vi "GPX_speed_test.vi"() -> ()   [LabVIEW 2017]
uses:
  <vilib>/Analysis/NI_AALPro.lvlib
panel:
  in  "GPX File Path":path
  out "acceleration graph":cluster{timestamp[], dbl[]}[](graph)
  out "acc Integral speed":dbl[](array[numeric])
  out "gps mean speed":dbl format="%0.2f"
  out "distance [m]":dbl
  in  "elotlás [s]":dbl
  in  "Eltol":bool
  out "delta t [s]":dbl
  in  "stop":bool
  in  "reset":bool
  in  "binary path (use dialog)":path
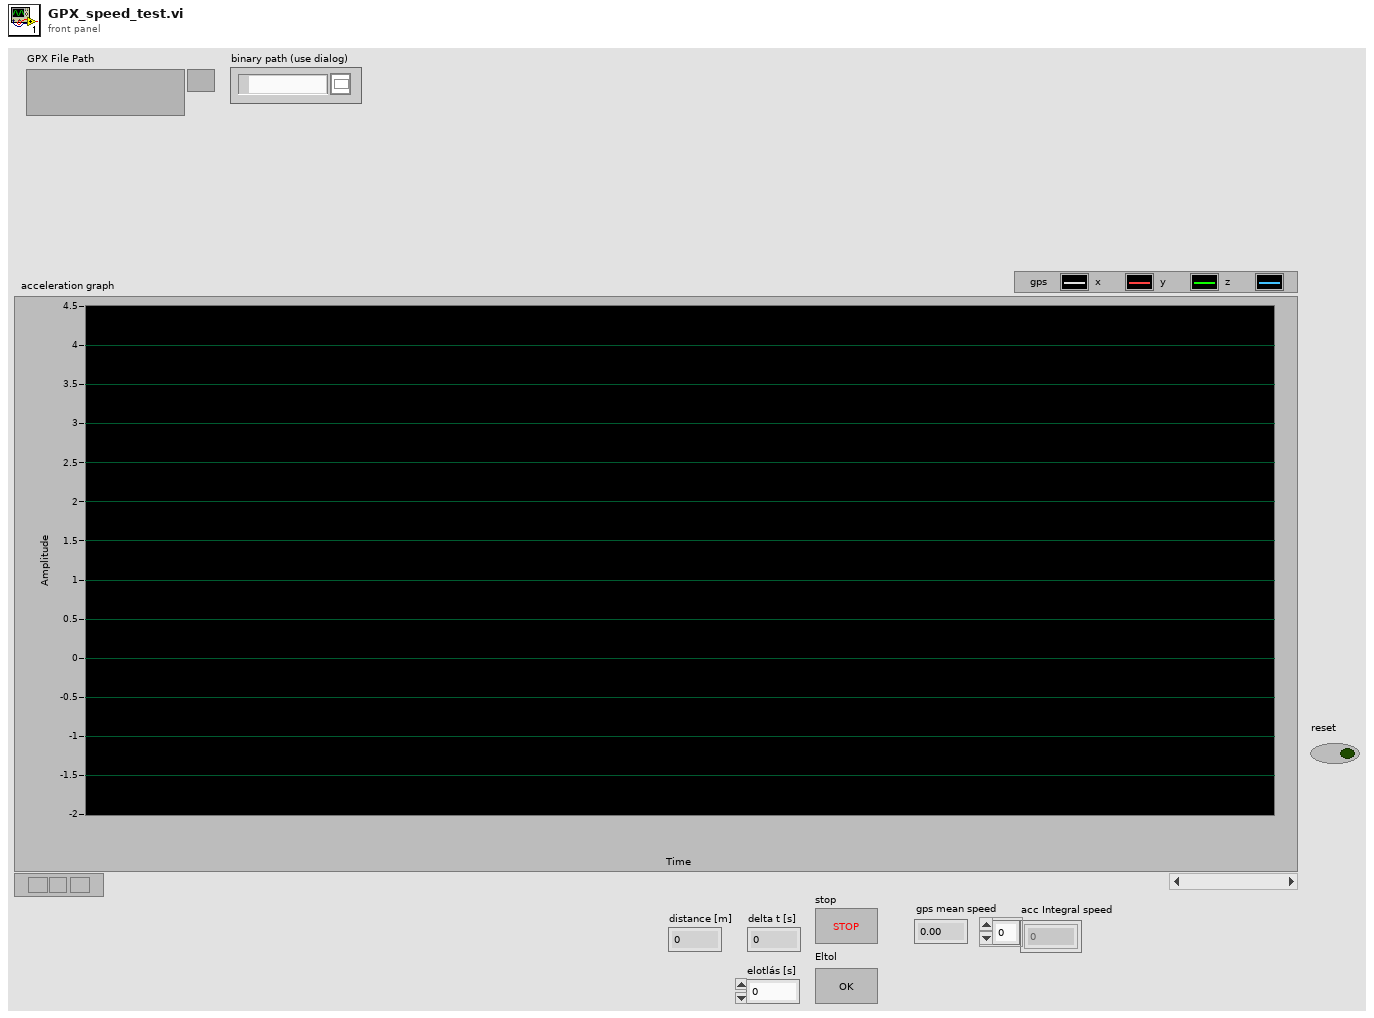
[diagram p1: front panel]
types:
  T1 = typedef "control_time_informations.ctl" = cluster{"starting time":timestamp, "ending time":timestamp, "dt[s]":dbl, "sampling rate [Hz]":dbl, "length":dbl}
  T2 = typedef "control_measurement_settings.ctl" = cluster{"sampling frequency [Hz]":dbl, "measurement interval [± g]":i32, "high precision?":bool, "number of pages":i32, "rate code":i32, "range code":i32, "id":i32}
  T3 = cluster{"statistics":cluster{"mean of x axis acceleration":dbl, "standard devation of x axis acceleration":dbl, "mean of y axis acceleration":dbl, "standard devation of y axis acceleration":dbl, "mean of z axis acceleration":dbl, "standard devation of z axis acceleration":dbl, "mean of magnitude of acceleration":dbl, "standard devation of magnitude of acceleration":dbl}, "time informations":T1, "actigraph settings":T2}
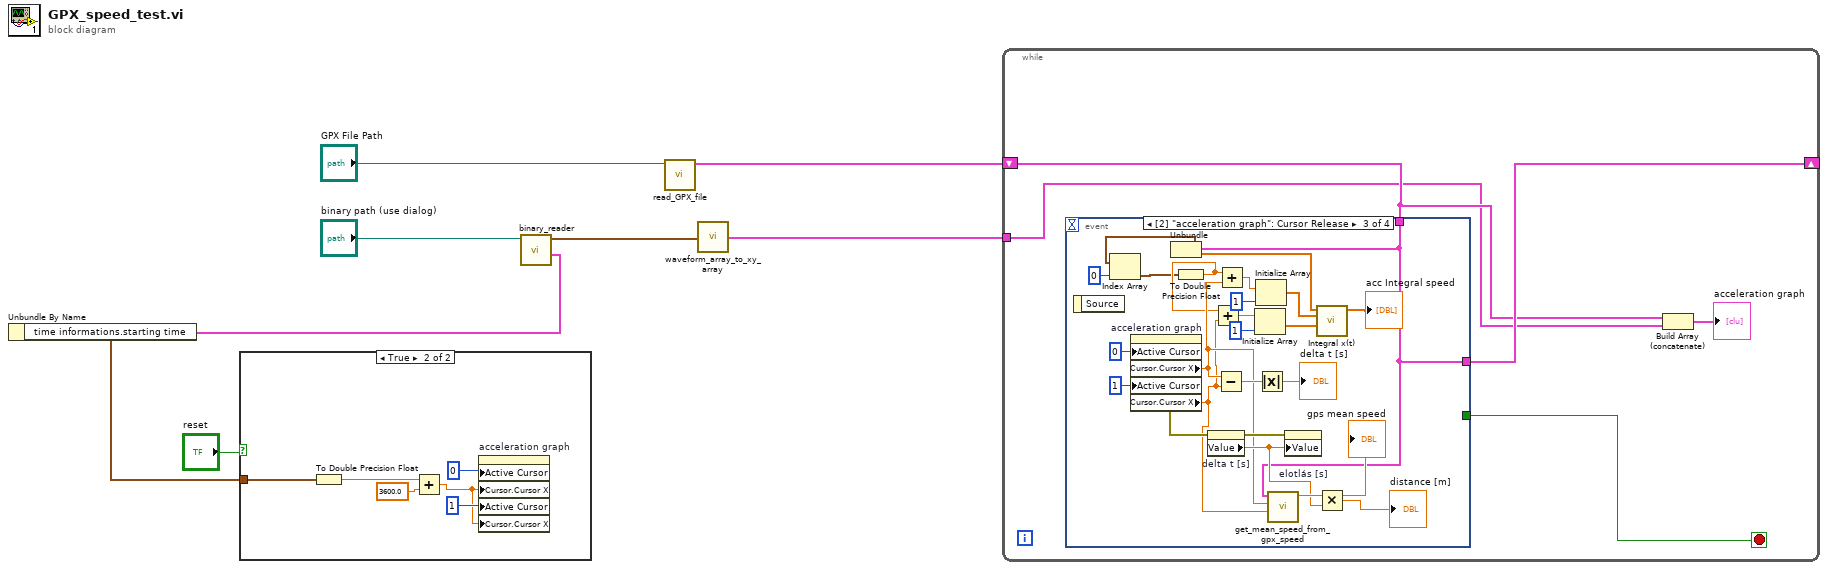
[diagram p0: block diagram]
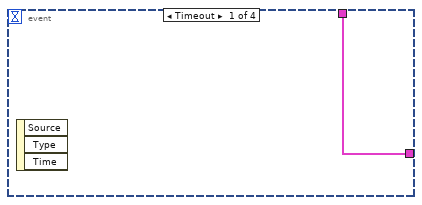
[diagram p2: hidden frame]
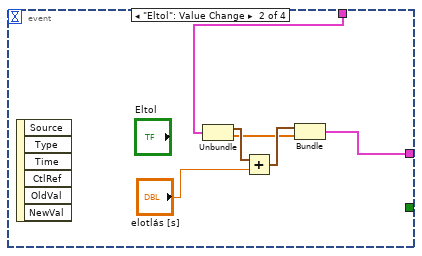
[diagram p3: hidden frame]
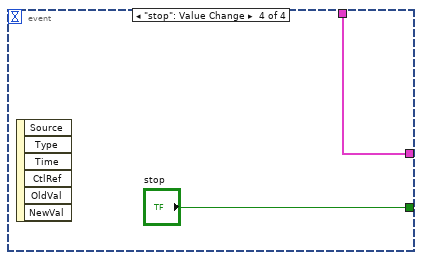
[diagram p4: hidden frame]
diagram:
  n1 = call "binary_reader.vi"("path to binary file"="binary path (use dialog)") -> ("Misc"=w6:T3, "3 axis acceleration in time"=w4:waveform(dbl)[])  [unwired: 6 in, 2 out]
  n2 = Unbundle By Name(w6) -> ("time informations.starting time"=w5:timestamp)
  n3 = case shown="True" "reset" {
    tunnel: w5 -> [_ w12]
    frame False {
    }
    frame True {
      n4 = To Double Precision Float(number=w12) -> (double precision float=w13:dbl)
      n5 = Add(x=w13, y=3600.0) -> (x+y=w9:dbl)
      n6 = property on="acceleration graph" class="XYGraph (strict)"("Active Cursor"=u32 0, "Cursor.Cursor X"=w9, "Active Cursor"=u32 1, "Cursor.Cursor X"=w9) -> ()  [unwired: 2 in, 2 out]
    }
  }
  n7 = call "read_GPX_file.vi"("GPX File Path"="GPX File Path") -> ("XY Speed data"=w2:cluster{timestamp[], dbl[]})  [unwired: 3 in, 3 out]
  n8 = call "waveform_array_to_xy_array.vi"("waveform array"=w4) -> ("XY array"=w3:cluster{timestamp[], "Y":dbl[]}[])
  n9 = while {
    shift-right: [w18] -> _
    shift-left: w2 -> [w17]
    tunnel: w3 -> [w15]
    stop <- w19 stop-if-true
    n10 = event shown="[2] \"acceleration graph\": Cursor Release" {
      selector: _ -> [_ _ _ _]
      dyn-events: _ -> [_ _ _ _]
      timeout: _ -> [_ _ _ _]
      tunnel: [_ _ _ "stop"] -> w19
      tunnel: [w20 w21 w30 w51] -> w18
      tunnel: w17 -> [w20 w25 w30 w51]
      event Timeout {
        n11 = event-data() -> ()  [unwired: 1 in, 3 out]
      }
      event "Eltol": Value Change {
        n12 = event-data() -> ()  [unwired: 1 in, 6 out]
        n13 = Unbundle(w25) -> (w24:timestamp[], w22:dbl[])
        n14 = Add(x=w24, y="elotlás [s]") -> (x+y=w23:timestamp[])
        n15 = Bundle(w23, w22) -> (w21:cluster{timestamp[], dbl[]})  [unwired: 1 in]
      }
      event "acceleration graph": Cursor Release {
        n16 = event-data() -> ()  [unwired: 1 in, 1 out]
        n17 = property on="acceleration graph" class="XYGraph (strict)"("Active Cursor"=u32 0, "Active Cursor"=u32 1) -> (error out=w47:errorcluster, "Cursor.Cursor X"=w36:dbl, "Cursor.Cursor X"=w32:dbl)  [unwired: 2 in, 1 out]
        n18 = Unbundle(w30) -> (w29:timestamp[], w27:dbl[])
        n19 = Index Array(array=w29, index=0) -> (element=w31:timestamp)
        n20 = To Double Precision Float(number=w31) -> (double precision float=w33:dbl)
        n21 = property on="delta t [s]" class="DigNum (strict)"(error in=w47) -> (error out=w46:errorcluster, "Value"=w43:dbl)  [unwired: 1 in, 1 out]
        n22 = Add(x=w33, y=w32) -> (x+y=w34:dbl)
        n23 = Subtract(x=w36, y=w32) -> (x-y=w50:dbl)
        n24 = Add(x=w33, y=w36) -> (x+y=w35:dbl)
        n25 = Initialize Array(w34, 1 ("dimension size")) -> (w39:dbl[])
        n26 = Initialize Array(w35, 1 ("dimension size")) -> (w42:dbl[])
        n27 = Absolute Value(x=w50) -> (abs(x)=→"delta t [s]":dbl)
        n28 = call "get_mean_speed_from_gpx_speed.vi"("to"=w32, "from"=w36, "speed"=w30) -> ("mean"=w45:dbl)  [unwired: 8 in]
        "gps mean speed" <- w45
        n29 = property on="elotlás [s]" class="DigNum (strict)"(error in=w46, "Value"=w43) -> ()  [unwired: 1 in, 2 out]
        n30 = call <vilib>:"Integral x(t).vi"("Final Condition"=w39, "Initial Condition"=w42, "X"=w27) -> ("Integral X"=→"acc Integral speed":dbl[])  [unwired: 7 in, 1 out]
        n31 = Multiply(x=w45, y=w43) -> (x*y=→"distance [m]":dbl)
      }
      event "stop": Value Change {
        n32 = event-data() -> ()  [unwired: 1 in, 6 out]
      }
    }
    n33 = Build Array (concatenate)(w17, w15) -> (→"acceleration graph":cluster{timestamp[], "Y":dbl[]}[])
  }
